vi "Test Animal Can Sleep after Eating.vi"(8 "error in (no error)":errorcluster, 11 "Animal Test In":refnum<class "Animal Test.lvclass">) -> (0 "error out":errorcluster, 3 "Animal Test Out":refnum<class "Animal Test.lvclass">)   [LabVIEW 2020, in "Animal Test.lvclass"]
doc: "Test Animal can sleep after eating"
uses:
  Animal Test.lvclass
  C:/git/astemes-lunit/source/API/LUnit Test Case/LUnit Test Case.lvclass
  Animal Test.lvclass/Animal Test.ctl
  API/LUnit Test Case/LUnit Test Case.lvclass/LUnit Test Case.ctl
  148b0b57-aa4b-4a32-929d-fe8f5b5d798f.vi
  API/LUnit Test Case/Private/Append Pass Result.vi
  API/LUnit Test Case/Private/Append Fail Result.vi
  API/LUnit Test Case/Private/Compare Variants.vi
  API/LUnit Test Case/Private/Describe Comparison.vi
  API/LUnit Test Case/Private/Variant to string.vi
  <vilib>/Utility/Data Type/Get Type Information.vi
  <vilib>/Utility/LVClass/Get LV Class Name.vi
  Animal Classes/Animal/Animal.lvclass
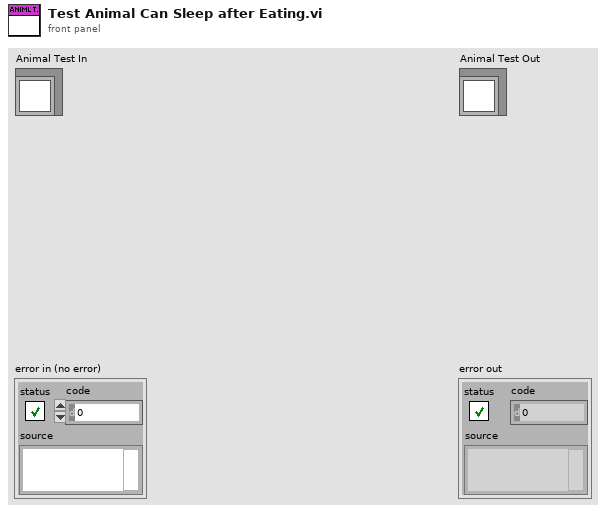
[diagram p1: front panel]
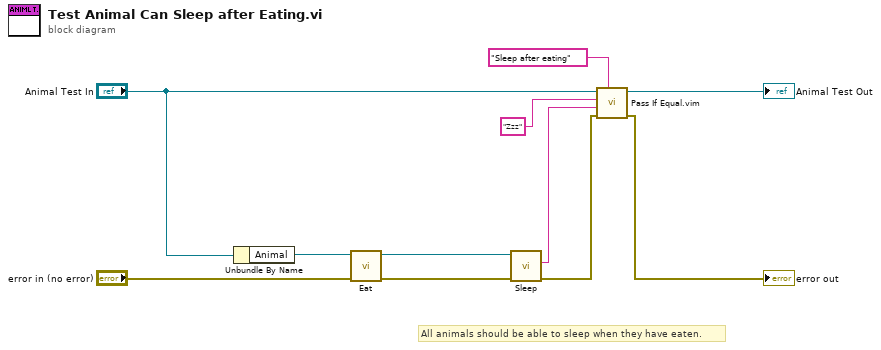
[diagram p0: block diagram]
diagram:
  # "All animals should be able to sleep when they have eaten."
  n1 = Unbundle By Name("Animal Test In") -> ("Animal"=w11:refnum<class "Animal.lvclass">)
  n2 = call-dynamic "Eat.vi"("error in (no error)"="error in (no error)", "Animal In"=w11) -> ("error out"=w2:errorcluster, "Animal Out"=w10:refnum<class "Animal.lvclass">)  [unwired: 7 in, 1 out]
  n3 = call-dynamic "Sleep.vi"("error in (no error)"=w2, "Animal in"=w10) -> ("error out"=w7:errorcluster, "Result"=w4:string)  [unwired: 7 in, 1 out]
  n4 = call "Pass If Equal.vim"("Description"="Sleep after eating", "error in (no error)"=w7, "Actual"=w4, "Expected"="Zzz" ("Result"), "LUnit Test Case In"="Animal Test In") -> ("error out"=→"error out":errorcluster, "LUnit Test Case Out"=→"Animal Test Out":refnum<class "Animal Test.lvclass">)  [unwired: 5 in]
